vi "finale.vi"() -> ()   [LabVIEW 2021]
uses:
  <vilib>/Instr/_visa.llb/VISA Configure Serial Port (Instr).vi
  <vilib>/addons/control/pid/pid.llb/PID (DBL).vi
  <vilib>/Utility/file.llb/Write Delimited Spreadsheet (DBL).vi
  <vilib>/addons/control/pid/NI_PID_pid.lvlib
panel:
  out "velocità":dbl
  out "Velocità":dbl(knob) scale=0.0..1300.0
  out "dt out (s)":dbl format="%.3f"
  in  "PWM.txt":path
  in  "data bits (8)":u16=8 min=5 max=8 step=1
  in  "baud rate (9600)":u32=9600
  in  "VISA resource name":refnum<visa-resource-name>
  in  "stop 2":bool
  out "Numero iterazioni":i32
  in  "setpoint":dbl format="%.2f"
  out "SP & PV":cluster{"initial PV":dbl, "SP:":dbl}(graph)
  in  "PID gains":T1={"proportional gain (Kc)"=1.0, "integral time (Ti, min)"=0.01, "derivative time (Td, min)"=0.0} {"derivative time (Td, min)" format="%.3f"; "integral time (Ti, min)" format="%.3f"; "proportional gain (Kc)" format="%.3f"}
  out "Thermometer":dbl(slide) scale=0.0..100.0
  in  "dt (s)":dbl=-1.0 format="%.3f"
  in  "output range":cluster{"output high":dbl, "output low":dbl}={"output high"=100.0, "output low"=-100.0} {"output low" format="%.2f"; "output high" format="%.2f"}
  out "PWM":dbl format="%.2f"
  out "MV":dbl(graph)
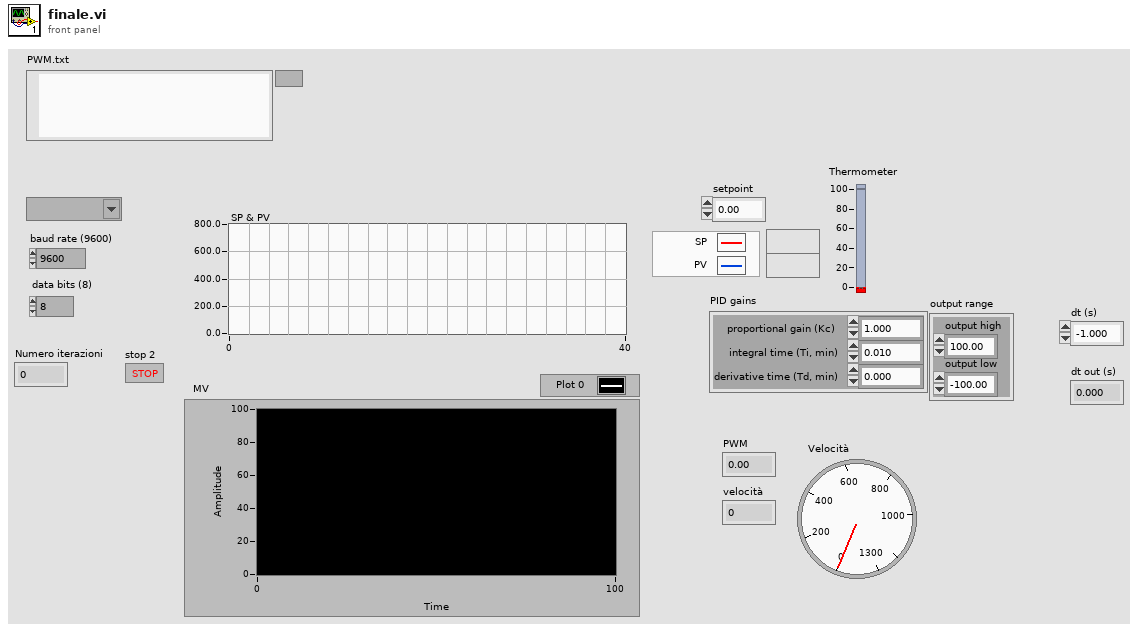
[diagram p1: front panel]
types:
  T1 = cluster{"proportional gain (Kc)":dbl, "integral time (Ti, min)":dbl, "derivative time (Td, min)":dbl}
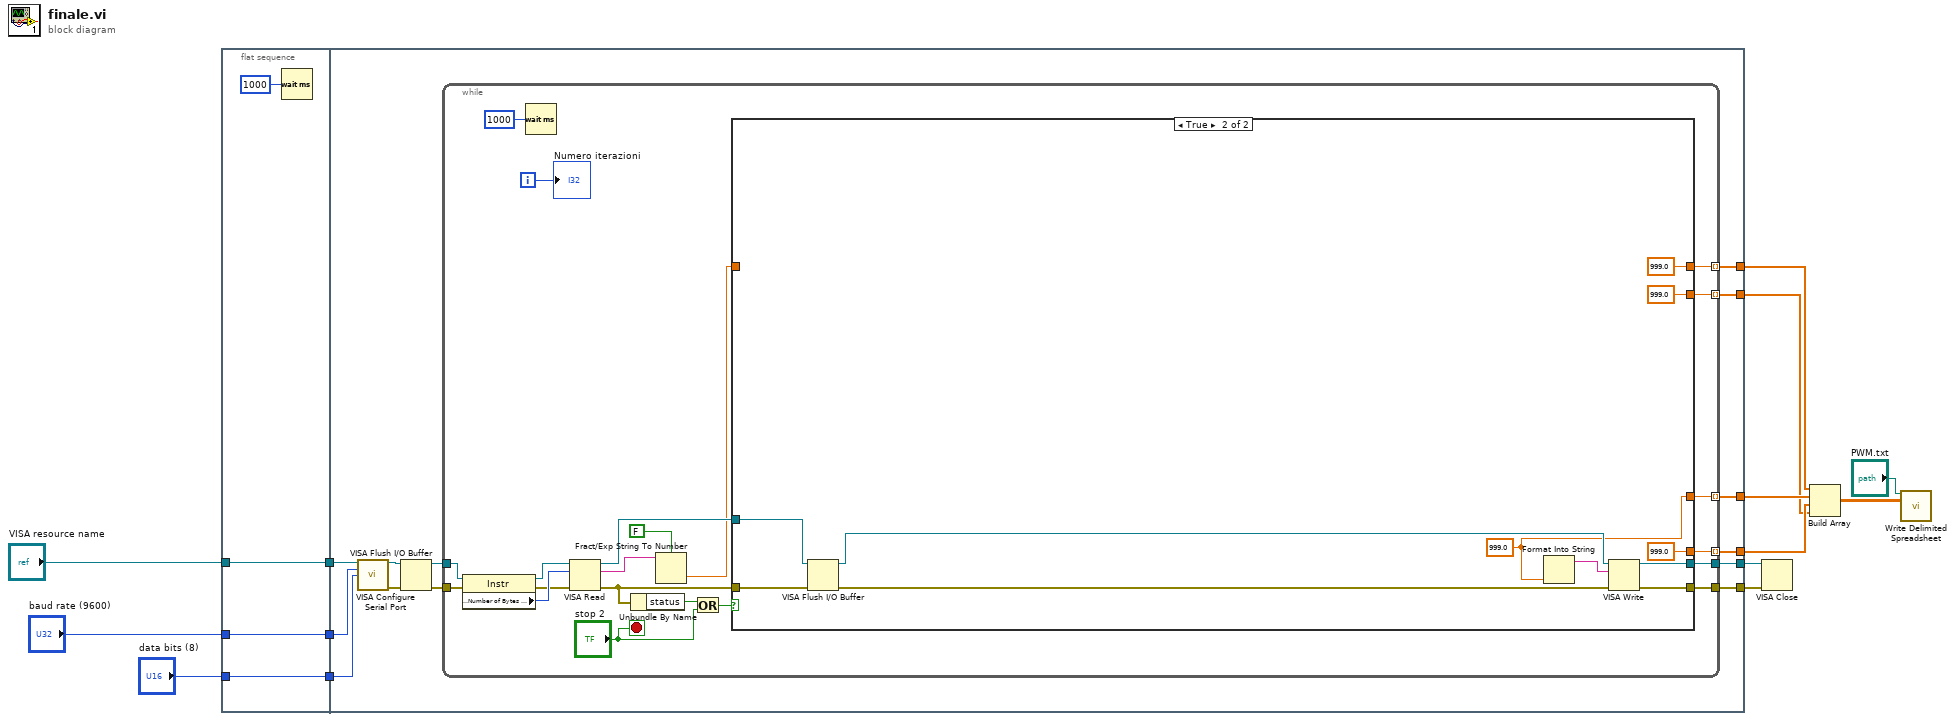
[diagram p0: block diagram]
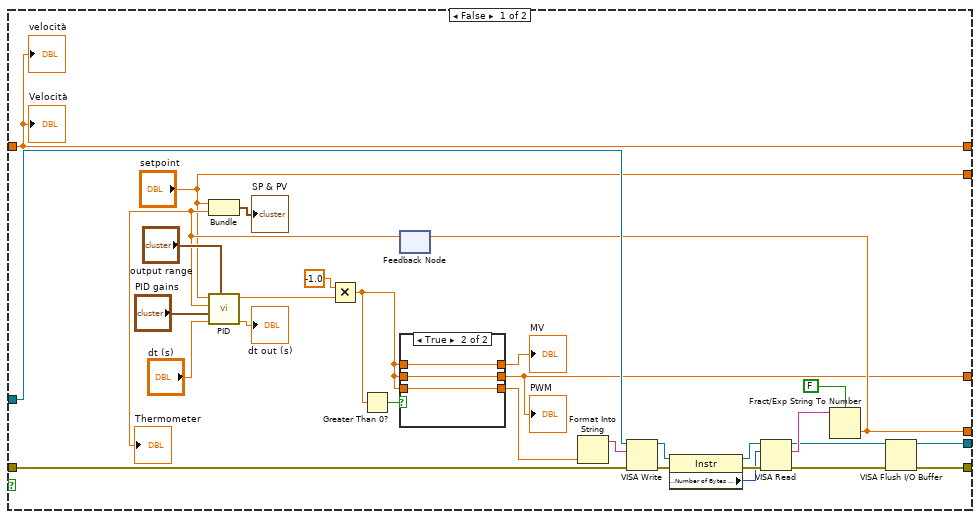
[diagram p2: hidden frame]
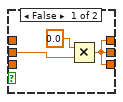
[diagram p3: hidden frame]
diagram:
  n1 = flat-sequence {
    tunnel: "baud rate (9600)" -> [w16]
    tunnel: "data bits (8)" -> [w17]
    tunnel: "VISA resource name" -> [w18]
    tunnel: [w18] -> w3
    tunnel: [w17] -> w2
    tunnel: [w16] -> w1
    tunnel: [w28] -> w10
    tunnel: [w27] -> w9
    tunnel: [w26] -> w7
    tunnel: [w25] -> w6
    tunnel: [w24] -> w5
    tunnel: [w23] -> w4
    tunnel: w3 -> [w29]
    tunnel: w2 -> [w30]
    tunnel: w1 -> [w31]
    frame #0 {
      n2 = Wait (ms)(milliseconds to wait=u32 1000) -> ()  [unwired: 1 out]
    }
    frame #1 {
      n3 = call-poly "VISA Configure Serial Port"("VISA resource name"=w29, "baud rate (9600)"=w31, "data bits (8)"=w30) -> ("VISA resource name out"=w19:refnum<visa-resource-name>, "error out"=w22:errorcluster)  [unwired: 11 in]
      n4 = VISA Flush I/O Buffer(VISA resource name=w19, error in (no error)=w22) -> (VISA resource name out=w21:refnum<visa-resource-name>, error out=w20:errorcluster)  [unwired: 1 in]
      n5 = while {
        tunnel: [w45] -> w27 mode=indexing
        tunnel: [w44] -> w28
        tunnel: [w43] -> w26
        tunnel: [w36] -> w25 mode=indexing
        tunnel: [w35] -> w24 mode=indexing
        tunnel: [w34] -> w23 mode=indexing
        tunnel: w21 -> [w33]
        tunnel: w20 -> [w32]
        i -> [w49]
        stop <- "stop 2" stop-if-true
        n6 = property class="Instr"(reference=w33, error in=w32) -> (reference out=w41:refnum<visa-resource-name>, error out=w40:errorcluster, "Serial Settings:Number of Bytes at Serial Port"=w42:u32)
        n7 = Wait (ms)(milliseconds to wait=u32 1000) -> ()  [unwired: 1 out]
        n8 = VISA Read(VISA resource name=w41, byte count=w42, error in (no error)=w40) -> (VISA resource name out=w39:refnum<visa-resource-name>, read buffer=w52:string, error out=w38:errorcluster)  [unwired: 1 out]
        n9 = Unbundle By Name(w38) -> ("status"=w51:bool)
        n10 = Fract/Exp String To Number(use system decimal point (T)=FALSE, string=w52) -> (number=w37:dbl)  [unwired: 2 in, 1 out]
        n11 = Or(x=w51, y="stop 2") -> (x .or. y?=w47:bool)
        n12 = case shown="True" w47 {
          tunnel: w38 -> [w79 w94]
          tunnel: w39 -> [w78 w95]
          tunnel: [w53 999.0 ("output")] -> w45
          tunnel: [w81 w98] -> w44
          tunnel: [w80 w97] -> w43
          tunnel: w37 -> [w53 _]
          tunnel: [w54 w90] -> w36
          tunnel: [w57 999.0] -> w35
          tunnel: ["setpoint" 999.0 ("setpoint")] -> w34
          frame False {
            n13 = feedback #1() -> (w58:dbl)  [unwired: 1 in]
            "Thermometer" <- w58
            n14 = Bundle("setpoint"="setpoint", w58) -> (→"SP & PV":cluster{"setpoint":dbl, dbl})  [unwired: 1 in]
            n15 = call-poly <vilib>:"PID.vi"("output range"="output range", "dt (s)"="dt (s)", "PID gains"="PID gains", "process variable"=w58, "setpoint"="setpoint") -> ("dt out (s)"=→"dt out (s)":dbl, "output"=w66:dbl)  [unwired: 5 in]
            n16 = Multiply(x=-1.0, y=w66) -> (x*y=w82:dbl)
            n17 = Greater Than 0?(x=w82) -> (x > 0?=w64:bool)
            n18 = case shown="True" w64 {
              tunnel: w82 -> [w85 w88]
              tunnel: [w83 w88] -> w54
              tunnel: [w83 w87] -> w69
              tunnel: w82 -> [_ w87]
              tunnel: [w83 w86] -> w65
              tunnel: w82 -> [_ w86]
              frame False {
                n19 = Multiply(x=0.0, y=w85) -> (x*y=w83:dbl)
              }
              frame True {
              }
            }
            "PWM" <- w54
            "MV" <- w65
            n20 = Format Into String(w69) -> (resulting string=w68:string)  [unwired: 3 in, 1 out]
            n21 = VISA Write(VISA resource name=w78, write buffer=w68, error in (no error)=w79) -> (VISA resource name out=w73:refnum<visa-resource-name>, error out=w72:errorcluster)  [unwired: 1 out]
            n22 = property class="Instr"(reference=w73, error in=w72) -> (reference out=w77:refnum<visa-resource-name>, error out=w76:errorcluster, "Serial Settings:Number of Bytes at Serial Port"=w75:u32)
            n23 = VISA Read(VISA resource name=w77, byte count=w75, error in (no error)=w76) -> (VISA resource name out=w70:refnum<visa-resource-name>, read buffer=w74:string, error out=w71:errorcluster)  [unwired: 1 out]
            n24 = Fract/Exp String To Number(use system decimal point (T)=FALSE, string=w74) -> (number=w57:dbl)  [unwired: 2 in, 1 out]
            n25 = feedback-in #1(w57) -> ()
            n26 = VISA Flush I/O Buffer(VISA resource name=w70, error in (no error)=w71) -> (VISA resource name out=w80:refnum<visa-resource-name>, error out=w81:errorcluster)  [unwired: 1 in]
            "Velocità" <- w53
            "velocità" <- w53
          }
          frame True {
            w90 = 999.0
            n27 = VISA Flush I/O Buffer(VISA resource name=w95, error in (no error)=w94) -> (VISA resource name out=w93:refnum<visa-resource-name>, error out=w92:errorcluster)  [unwired: 1 in]
            n28 = Format Into String(w90) -> (resulting string=w89:string)  [unwired: 3 in, 1 out]
            n29 = VISA Write(VISA resource name=w93, write buffer=w89, error in (no error)=w92) -> (VISA resource name out=w97:refnum<visa-resource-name>, error out=w98:errorcluster)  [unwired: 1 out]
          }
        }
        "Numero iterazioni" <- w49
      }
    }
  }
  n30 = VISA Close(VISA resource name=w7, error in (no error)=w10) -> ()  [unwired: 1 out]
  n31 = Build Array(w9, w6, w5, w4) -> (w8:dbl[][])
  n32 = call-poly <vilib>:"Write Delimited Spreadsheet.vi"("file path (dialog if empty)"="PWM.txt", "2D data"=w8) -> ()  [unwired: 12 in, 2 out]
